vi "Motion_Close.vi"(8 "error in (no error)":errorcluster, 11 "connection ID":refnum<k5>) -> (0 "error out":errorcluster)   [LabVIEW 2010]
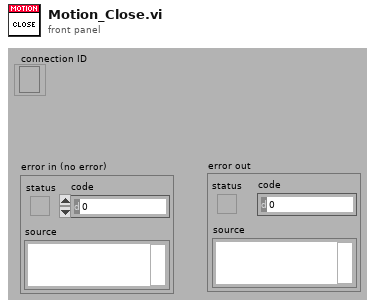
[diagram p1: front panel]
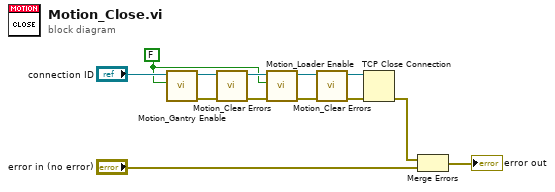
[diagram p0: block diagram]
diagram:
  w1 = FALSE ("Enable? (T)")
  n1 = call "Motion_Gantry Enable.vi"("Enable? (T)"=w1, "TCP Connection Refnum in"="connection ID") -> ("error out"=w12:errorcluster, "TCP Connection Refnum (dup)"=w11:refnum<k5>)  [unwired: 8 in]
  n2 = call "Motion_Clear Errors.vi"("error in (no error)"=w12, "TCP Connection Refnum in"=w11) -> ("error out"=w6:errorcluster, "TCP Connection Refnum (dup)"=w7:refnum<k5>)  [unwired: 8 in]
  n3 = call "Motion_Loader Enable.vi"("error in (no error)"=w6, "Enable? (T)"=w1, "TCP Connection Refnum in"=w7) -> ("error out"=w4:errorcluster, "TCP Connection Refnum (dup)"=w5:refnum<k5>)  [unwired: 7 in]
  n4 = call "Motion_Clear Errors.vi"("error in (no error)"=w4, "TCP Connection Refnum in"=w5) -> ("error out"=w2:errorcluster, "TCP Connection Refnum (dup)"=w3:refnum<k5>)  [unwired: 8 in]
  n5 = TCP Close Connection(connection ID=w3, error in (no error)=w2) -> (error out=w10:errorcluster)  [unwired: 1 in, 1 out]
  n6 = Merge Errors(w10, "error in (no error)") -> (→"error out":errorcluster)
